vi "Get Path to VI Under Test.vi"(8 "error in (no error)":errorcluster, 10 "LVTest file":path, 11 "LUnit Test Vector in":refnum<class "LUnit Test Vector.lvclass">) -> (0 "error out":errorcluster, 3 "LUnit Test Vector out":refnum<class "LUnit Test Vector.lvclass">)   [LabVIEW 2020, in "LUnit Test Vector.lvclass"]
uses:
  LUnit Test Vector.lvclass
  LUnit Test Vector.lvclass/LUnit Test Vector.ctl
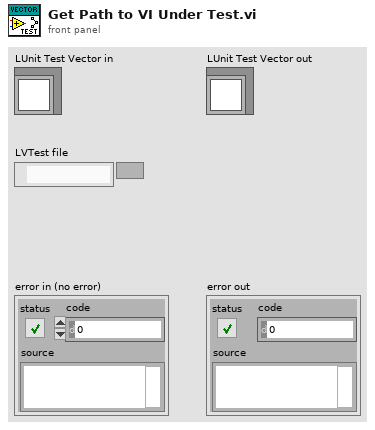
[diagram p1: front panel]
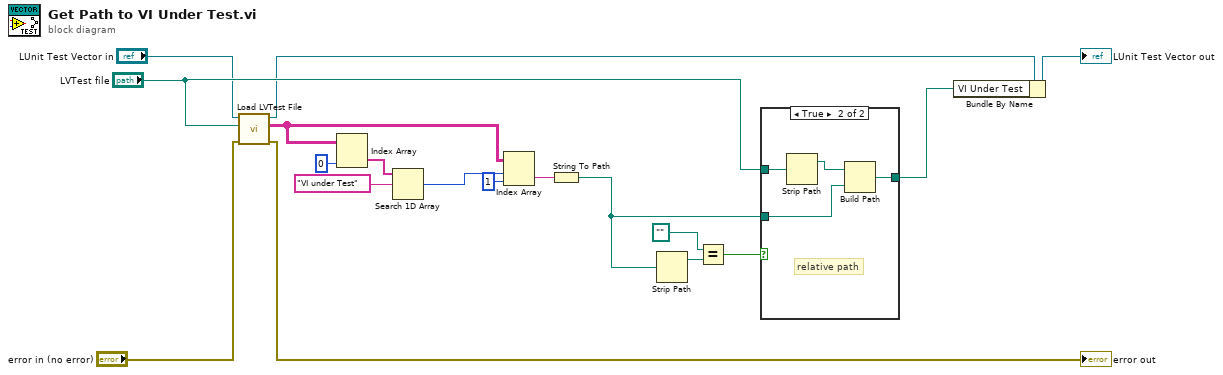
[diagram p0: block diagram]
diagram:
  n1 = call "Load LVTest File.vi"("error in (no error)"="error in (no error)", "LVTest file"="LVTest file", "LUnit Test Vector In"="LUnit Test Vector in") -> ("error out"=→"error out":errorcluster, "File Contents"=w6:string[][], "LUnit Test Vector Out"=w3:refnum<class "LUnit Test Vector.lvclass">)  [unwired: 5 in, 1 out]
  n2 = Index Array(array=w6, index (col)=0 ("disabled index (col)")) -> (element=w17:string[])  [unwired: 1 in]
  n3 = Search 1D Array(1D array=w17, element="VI under Test") -> (index of element=w15:i32)  [unwired: 1 in]
  n4 = Index Array(array=w6, index (row)=w15, index (col)=1 ("disabled index (col)")) -> (element=w13:string)
  n5 = String To Path(string=w13) -> (path=w7:path)
  n6 = Strip Path(path=w7) -> (stripped path=w11:path)  [unwired: 1 out]
  n7 = Equal?(x=path "" ("stripped path"), y=w11) -> (x = y?=w9:bool)
  n8 = case shown="True" w9 {
    tunnel: [w19 w23] -> w8
    tunnel: w7 -> [w19 w22]
    tunnel: "LVTest file" -> [_ w20]
    frame False {
      # "absolute path"
    }
    frame True {
      # "relative path"
      n9 = Strip Path(path=w20) -> (stripped path=w21:path)  [unwired: 1 out]
      n10 = Build Path(base path=w21, name or relative path=w22) -> (appended path=w23:path)
    }
  }
  n11 = Bundle By Name(cluster=w3, "VI Under Test"=w8) -> (→"LUnit Test Vector out":refnum<class "LUnit Test Vector.lvclass">)
